vi "Data to LV BMS Status.vi"(1 "Data":u8[](array[numeric])) -> (0 "BMS Low Voltage Status":T1 {"Temp. 0" scale=0.0..100.0; "Temp. 1" scale=0.0..100.0})   [LabVIEW 2016]
uses:
  BMS Voltage status 2.ctl
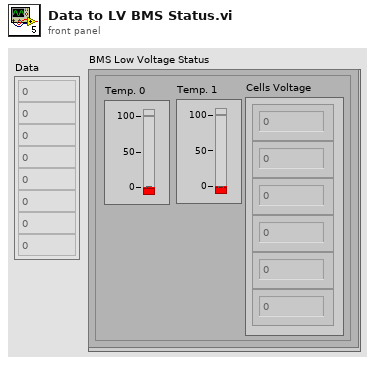
[diagram p1: front panel]
types:
  T1 = typedef "BMS Voltage status 2.ctl" = cluster{"Cells Voltage":dbl[], "Temp. 1":u8, "Temp. 0":u8}
  T2 = cluster{"Data[0]":u8, "Data[1]":u8, "Data[2]":u8, "Data[3]":u8, "Data[4]":u8, "Data[5]":u8, "Data[6]":u8, "Data[7]":u8, "Data[8]":u8}
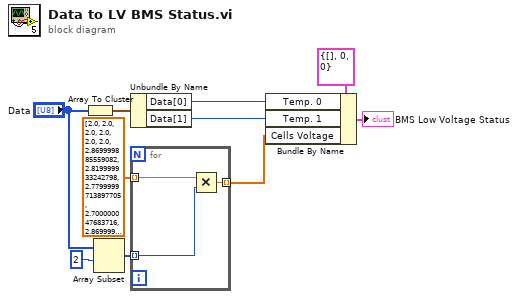
[diagram p0: block diagram]
diagram:
  n1 = Array To Cluster(array="Data") -> (cluster=w3:T2)
  n2 = Array Subset(array="Data", index=2) -> (w5:u8[])  [unwired: 1 in]
  n3 = Unbundle By Name(w3) -> ("Data[0]"=w2:u8, "Data[1]"=w1:u8)
  n4 = for {
    tunnel: sgl[] [2.0, 2.0, 2.0, 2.0, 2.0, 2.0, 2.87, 2.82, 2.78, 2.7, 2.87, 2.98] ("Data") -> [w13] mode=indexing
    tunnel: [w12] -> w8 mode=indexing
    tunnel: w5 -> [w11] mode=indexing
    n5 = Multiply(x=w13, y=w11) -> (x*y=w12:sgl)
  }
  n6 = Bundle By Name(cluster=T1 {"Cells Voltage"=[], "Temp. 1"=0, "Temp. 0"=0} ("BMS Low Voltage Status 2"), "Temp. 0"=w2, "Temp. 1"=w1, "Cells Voltage"=w8) -> (→"BMS Low Voltage Status":T1)
